vi "formatCfmToString.vi"(8 "error in (no error)":errorcluster, 9 "CFM 1":dynamicdata(waveform), 10 "CFM 2":dynamicdata(waveform), 11 "CFM 3":dynamicdata(waveform)) -> (0 "error out":errorcluster, 3 "String":string)   [LabVIEW 2019]
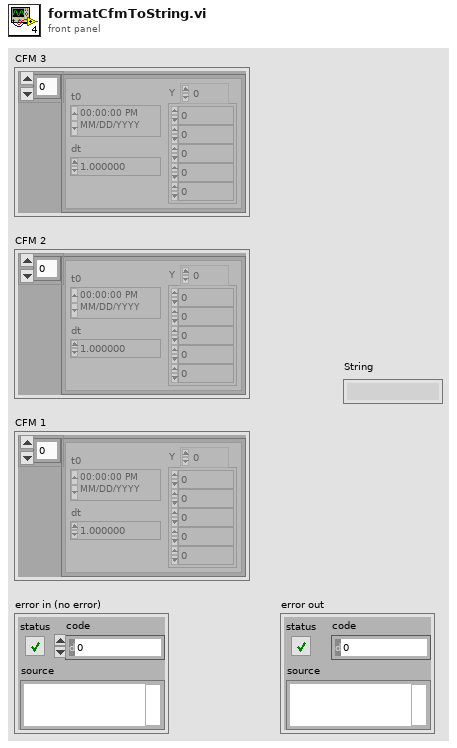
[diagram p1: front panel]
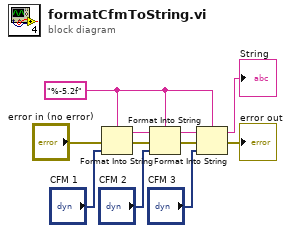
[diagram p0: block diagram]
diagram:
  w10 = "%-5.2f" ("format string")
  n1 = Format Into String(format string=w10, error in="error in (no error)", "CFM 1") -> (resulting string=w7:string, error out=w8:errorcluster)  [unwired: 1 in]
  n2 = Format Into String(format string=w10, initial string=w7, error in=w8, "CFM 2") -> (resulting string=w6:string, error out=w9:errorcluster)
  n3 = Format Into String(format string=w10, initial string=w6, error in=w9, "CFM 3") -> (resulting string=→"String":string, error out=→"error out":errorcluster)
